vi "LDA_Beam_Alignment.vi"() -> ()   [LabVIEW 2010]
uses:
  Anemometry Sub Vis/Controls/Beam_Type.ctl
  Anemometry Sub Vis/Gen Trav/Traverse_cluster.ctl
  Anemometry Sub Vis/Gen Trav/Spacing.ctl
  Anemometry Sub Vis/Controls/Multi_run_mode.ctl
  Anemometry Sub Vis/Controls/User_Specific_mode.ctl
  Anemometry Sub Vis/Controls/Post_Process.ctl
  Anemometry Sub Vis/Controls/Tunnel_Coordinates.ctl
  Anemometry Sub Vis/Gen Trav/Trav_mode.ctl
  Anemometry Sub Vis/Globals/Trav_pos_global.vi
  Anemometry Sub Vis/Globals/Meas_global.vi
  Anemometry Sub Vis/Globals/Preference_global.vi
panel:
  in  "Beams to peak":bool[](array[boolean])=[TRUE, TRUE, TRUE, TRUE]
  out "Beam Names":string[](array[string])
  out "Probe is facing...":string
  out "In-Plane Roll (deg)":dbl
  out "Pitch (deg)":dbl
  out "Yaw (deg)":dbl
  out "Vp (Actual Probe dir. vect)":dbl[](array[numeric])
  in  "Mode":T1(ring)
  out "Values Out":dbl[][](array[numeric]) format="%.2f"
  out "Original Position":dbl[](array[numeric]) format="%.2f"
  in  "Traverse Position":dbl[](array[numeric])=[0.0, 0.0, 0.0] format="%.2f"
  out "Message":string
  in  "Go Back":bool
  in  "OK":bool
  in  "stop":bool
  in  "Working On":T2 items=["Green Unshifted", "Green Shifted", "Blue Unshifted", "Blue Shifted"]
  # "X                 Y              Z"
  # "X                 Y              Z          Power"
  # "Green Unshifted\nGreen Shifted\nBlue Unshifted\nBlue Shifted"
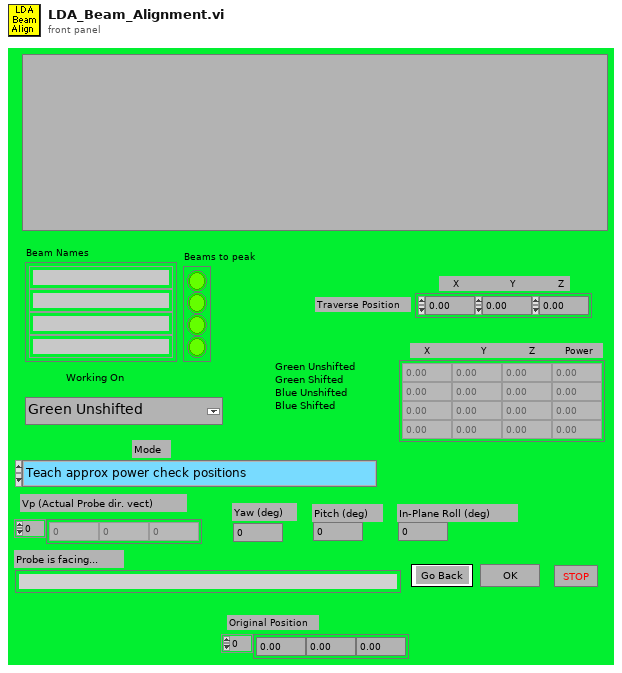
[diagram p1: front panel]
types:
  T1 = enum16{"Teach approx power check positions", "Hunt for optimum power check positions", "Check Beam powers now", "Peak up beam power using manipulators"}
  T2 = typedef "Beam_Type.ctl" = u16
  T3 = typedef "Traverse_cluster.ctl" = cluster{"Start X":dbl, "Start Y":dbl, "Start Z":dbl, "End X":dbl, "End Y":dbl, "End Z":dbl, "No. of pts.":i32, "Spacing":T4, "Filename":path, "Tunnel Speed":dbl, "Averaging time (min)":dbl, "Extra Commands":string, "Specific Arguments":string, "Emission Rate (l/min)":dbl, "Trace Gas Concentration (%)":dbl, "Density Ratio":string, "Comments":string, "Row No":i32, "Row Type Selector":T5, "Completion time":string, "Row Duration (mins)":dbl, "No. of Valid pts.":i32, "Meas Setup File":string}
  T4 = typedef "Spacing.ctl" = enum16{"Linear", "Log", "Gauss", "Specified", "N/A"}
  T5 = typedef "Multi_run_mode.ctl" = enum16{"Move Traverse Only", "Set Tunnel Speed Only", "Set Source Only", "Set Measurement Conditions", "Single Measurement", "Vertical Profile", "Lateral Profile", "Longitudinal Profile", "Explore Volume", "Multi-Axis Profile", "Auto Calibrate", "Meas Fast FID Bkgnd", "Check Beam Power", "Scanning Valve Measurement", "Run VI Named:", "Set ADAM Ch", "Wait (minutes)", "Send Message", "Synchronize With:", "Fall Back to this Row", "Turn Off Row Repeating", "Blank Row"}
  T6 = typedef "Tunnel_Coordinates.ctl" = enum16{"Work in Tunnel Coordinates", "Work in Model Coordinates"}
  T7 = typedef "User_Specific_mode.ctl" = enum16{"Check VI only", "Run VI"}
  T8 = typedef "Post_Process.ctl" = enum16{"Take New Data", "Post Process Raw Data File"}
  T9 = enum16{"Load setup from excel file", "Save setup to excel file"}
  T10 = enum16{"Load From Excel File", "Save to Excel File"}
  T11 = typedef "Trav_mode.ctl" = enum16{"Move traverse", "Read traverse position", "Teach Position"}
  T12 = typedef "LDA_Beam_Cluster.ctl" = cluster{"Vg1 (Green 1 dir. vect.)":dbl[], "Vg2  (Green 2 dir. vect.)":dbl[], "Vb1 (Blue 1 dir. vect.)":dbl[], "Vb2 (Blue 1 dir. vect.)":dbl[], "Porb (Orb XYZ posn. forced coplanar)":dbl[], "Porb (Orb XYZ posn. - allow skew)":dbl[], "Orb posn. uncertainty, +/- dx, dy, dz":dbl[], "Vp (Actual Probe dir. vect)":dbl[], "Yaw (deg)":dbl, "Pitch (deg)":dbl, "In-Plane Roll (deg)":dbl, "Beam Half Angle (deg)":dbl, "B1 Close P11":dbl[], "B1 Far P12":dbl[], "B2 Close P22":dbl[], "B2 Far P21":dbl[], "Projected Roll (deg)":dbl, "Green Velocity Vector":dbl[], "Blue Velocity Vector":dbl[], "Probe is facing....":string, "Calculation Method":string}
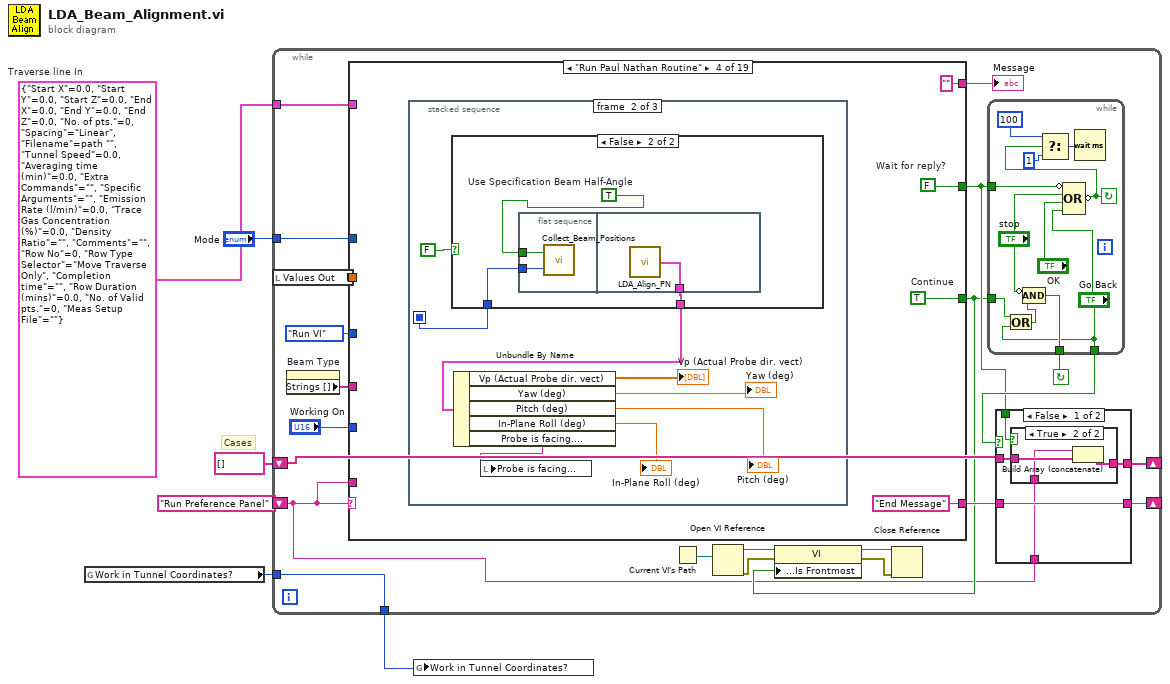
[diagram p0: block diagram]
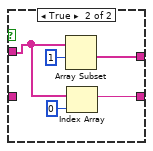
[diagram p3: hidden frame]
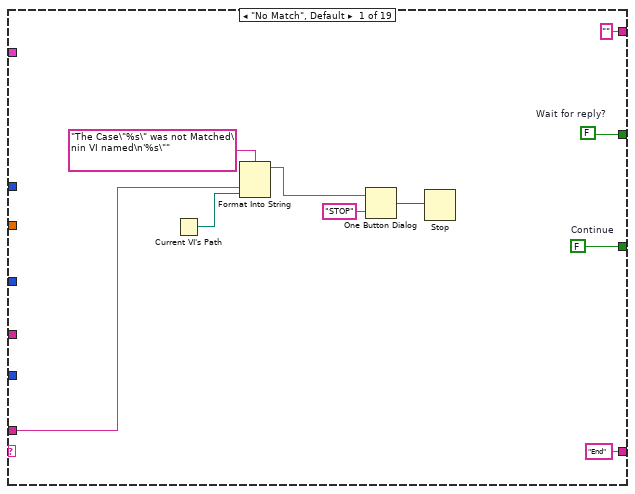
[diagram p4: hidden frame]
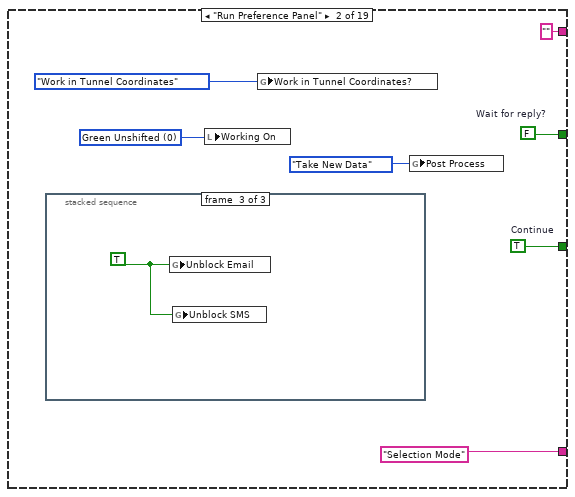
[diagram p5: hidden frame]
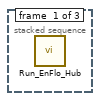
[diagram p6: hidden frame]
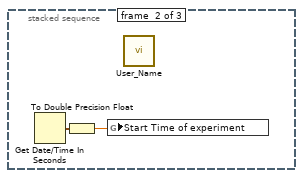
[diagram p7: hidden frame]
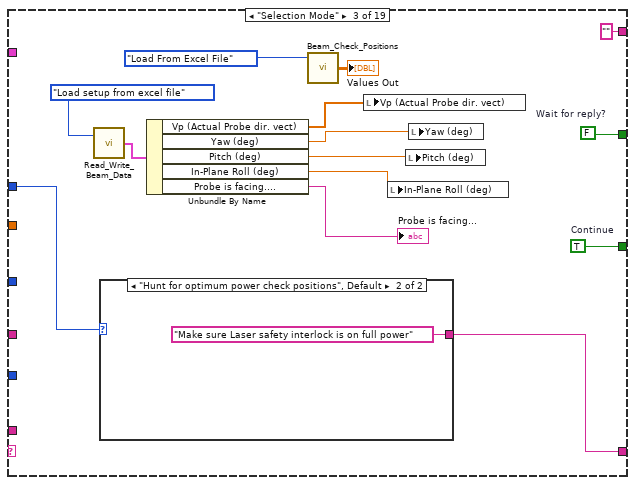
[diagram p8: hidden frame]
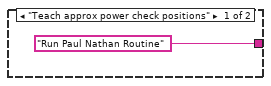
[diagram p9: hidden frame]
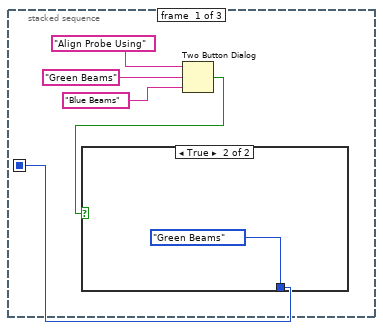
[diagram p10: hidden frame]
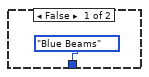
[diagram p11: hidden frame]
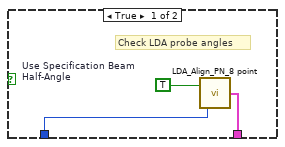
[diagram p12: hidden frame]
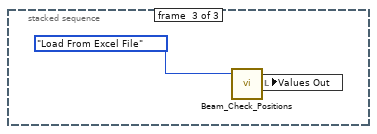
[diagram p13: hidden frame]
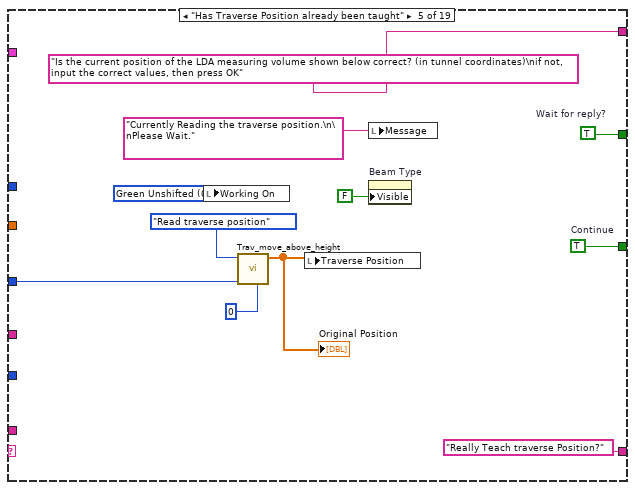
[diagram p14: hidden frame]
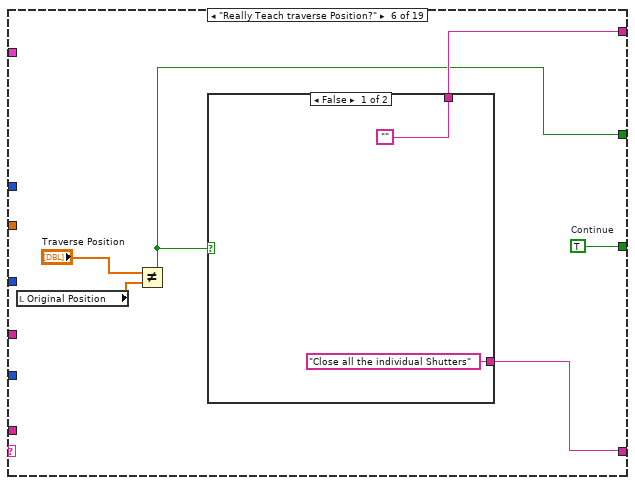
[diagram p15: hidden frame]
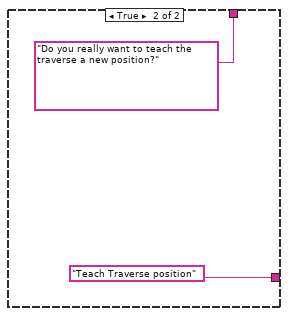
[diagram p16: hidden frame]
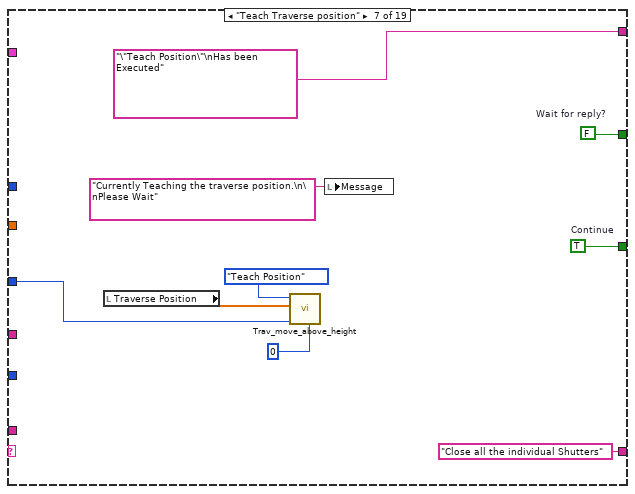
[diagram p17: hidden frame]
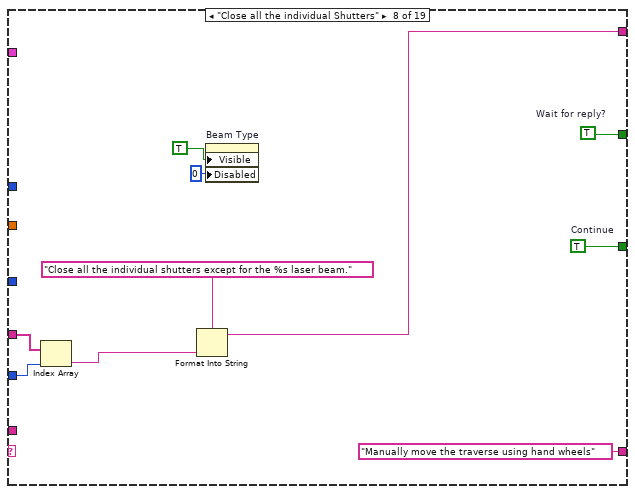
[diagram p18: hidden frame]
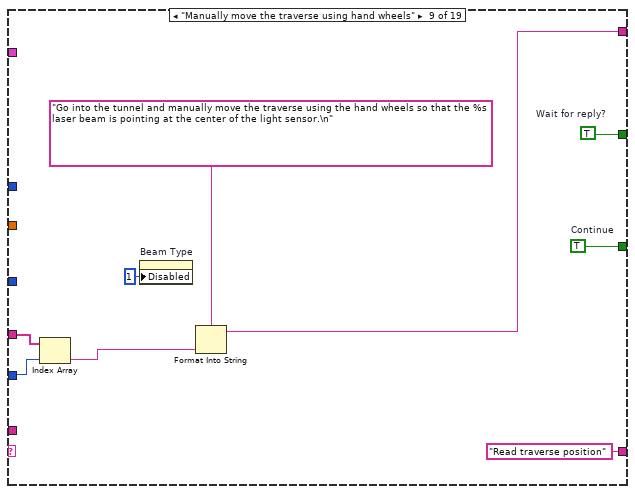
[diagram p19: hidden frame]
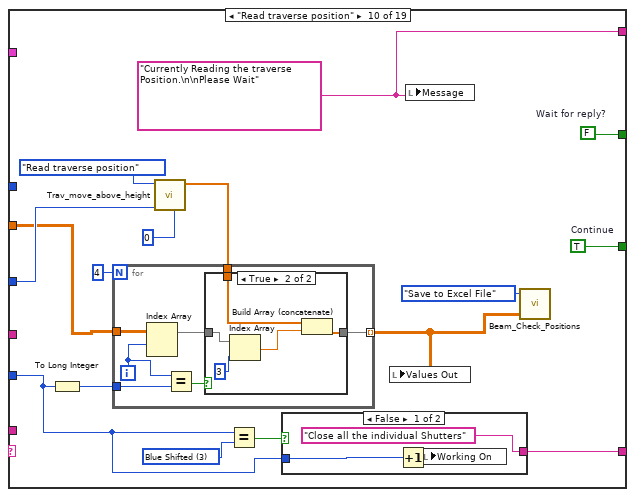
[diagram p20: hidden frame]
diagram:
  w3 = T3 {"Start X"=0.0, "Start Y"=0.0, "Start Z"=0.0, "End X"=0.0, "End Y"=0.0, "End Z"=0.0, "No. of pts."=0, "Spacing"=enum."Linear", "Filename"=path "", "Tunnel Speed"=0.0, "Averaging time (min)"=0.0, "Extra Commands"="", "Specific Arguments"="", "Emission Rate (l/min)"=0.0, "Trace Gas Concentration (%)"=0.0, "Density Ratio"="", "Comments"="", "Row No"=0, "Row Type Selector"=enum."Move Traverse Only", "Completion time"="", "Row Duration (mins)"=0.0, "No. of Valid pts."=0, "Meas Setup File"=""}  # Traverse line In
  # "Cases"
  n1 = global read "Trav_pos_global.vi" "Work in Tunnel Coordinates?"() -> (w1:T6)
  n2 = while {
    tunnel: w3 -> [w9]
    tunnel: "Mode" -> [w10]
    shift-left: string[] [] -> [w26]
    shift-right: [w25] -> _
    shift-left: "Run Preference Panel" -> [w8]
    shift-right: [w24] -> _
    tunnel: [w7] -> w2
    tunnel: w1 -> [w7]
    stop <- w28 continue-if-true
    n3 = local read "Values Out"() -> (w11:dbl[][])
    n4 = property on="Beam Type" class="Ring (strict)"() -> ("Strings []"=w13:string[])  [unwired: 2 in, 2 out]
    n5 = case shown="\"Run Paul Nathan Routine\"" w8 {
      tunnel: [w63 w70 w87 w93 w130 w136 w149 w159 w168 w184 w209 w219 w233 w259 w279 w283 w298 w306 w316] -> w14
      tunnel: ["End" "Selection Mode" w83 "End Message" "Really Teach traverse Position?" w131 "Close all the individual Shutters" "Manually move the traverse using hand wheels" "Read traverse position" w172 w203 "Hunt for optimum power check positions" "End Message" "End Message" "Read Beam Power" "Save measured beam Power" w290 "End Message" "End"] -> w23
      tunnel: [w62 w69 w86 w92 w129 w132 w148 w158 w167 w183 w208 w218 w234 w260 w278 w282 w297 w305 w315] -> w15
      tunnel: ["" "" "" "" "Is the current position of the LDA measuring volume shown below correct? (in tunnel coordinates)\nif not, input the correct values, then press OK" w135 "\"Teach Position\"\nHas been Executed" w152 w161 w169 "Make sure the Laser safety interlock is on full power and all the shutters are open." "Please select which beams you would like to hunt for optimum power check positions for by pressing the green buttons." "" "" w265 w281 w289 "Now open all the individual shutters so all four beam are showing." w309] -> w22
      tunnel: User_Specific_mode."Run VI" ("Simulate/Run") -> [_ _ _ _ w125 _ w144 _ _ w180 _ _ _ _ w275 _ _ _ _]
      tunnel: w13 -> [_ _ _ _ _ _ _ w157 w164 _ w206 w214 w222 _ w270 _ w286 _ _]
      tunnel: "Working On" -> [_ _ _ _ _ _ _ w156 w163 w171 w205 _ _ _ w269 _ w287 _ _]
      tunnel: w11 -> [_ _ _ _ _ _ _ _ _ w170 _ _ _ _ w268 _ w295 _ _]
      tunnel: w10 -> [_ _ w84 _ _ _ _ _ _ _ w204 _ _ _ _ _ _ _ w312]
      tunnel: w9 -> [_ _ _ _ _ _ _ _ _ _ _ _ _ w257 _ _ _ _ _]
      tunnel: w8 -> [w54 _ _ _ _ _ _ _ _ _ _ _ _ _ _ _ _ _ _]
      frame "No Match", Default {
        w62 = FALSE  # Wait for reply?
        w63 = FALSE  # Continue
        n6 = Current VI's Path() -> (path=w55:path)
        n7 = Format Into String(format string="The Case\"%s\" was not Matched\nin VI named\n'%s\"" ("Format String"), w54, w55) -> (resulting string=w58:string)  [unwired: 2 in, 1 out]
        n8 = One Button Dialog(message=w58, button name ("OK")="STOP") -> (true=w56:bool)
        n9 = Stop(stop? (T)=w56) -> ()
      }
      frame "Run Preference Panel" {
        w67 = T2 0 items=["Green Unshifted", "Green Shifted", "Blue Unshifted", "Blue Shifted"] ("Beam Type")
        w69 = FALSE  # Wait for reply?
        w70 = TRUE  # Continue
        n10 = stacked-sequence {
          frame #0 {
            n11 = call "Run_EnFlo_Hub.vi"() -> ()  [unwired: 8 out]
          }
          frame #1 {
            n12 = Get Date/Time In Seconds() -> (seconds since 1Jan1904=w72:timestamp)
            n13 = To Double Precision Float(number=w72) -> (double precision float=w71:dbl)
            n14 = global write "Meas_global.vi" "Start Time of experiment"(w71) -> ()
            n15 = call "User_Name.vi"() -> ()  [unwired: 1 out]
          }
          frame #2 {
            w73 = TRUE
            n16 = global write "Preference_global.vi" "Unblock Email"(w73) -> ()
            n17 = global write "Preference_global.vi" "Unblock SMS"(w73) -> ()
          }
        }
        n18 = local write "Working On"(w67) -> ()
        n19 = global write "Trav_pos_global.vi" "Work in Tunnel Coordinates?"(Tunnel_Coordinates."Work in Tunnel Coordinates" ("Work in Tunnel Coordinates?")) -> ()
        n20 = global write "Meas_global.vi" "Post Process"(Post_Process."Take New Data" ("Post Process")) -> ()
      }
      frame "Selection Mode" {
        w86 = FALSE  # Wait for reply?
        w87 = TRUE  # Continue
        n21 = call "Read_Write_Beam_Data.vi"("Mode"=T9."Load setup from excel file") -> ("Beam Data Out"=w75:T12)  [unwired: 1 in]
        n22 = case shown="\"Hunt for optimum power check positions\", Default" w84 {
          tunnel: ["Run Paul Nathan Routine" "Make sure Laser safety interlock is on full power"] -> w83
          frame "Teach approx power check positions" {
          }
          frame "Hunt for optimum power check positions", Default {
          }
        }
        n23 = Unbundle By Name(w75) -> ("Vp (Actual Probe dir. vect)"=w80:dbl[], "Yaw (deg)"=w77:dbl, "Pitch (deg)"=w78:dbl, "In-Plane Roll (deg)"=w79:dbl, "Probe is facing...."=→"Probe is facing...":string)
        n24 = call "Beam_Check_Positions.vi"("Mode"=T10."Load From Excel File") -> ("Values Out"=→"Values Out":dbl[][])  [unwired: 1 in, 1 out]
        n25 = local write "Vp (Actual Probe dir. vect)"(w80) -> ()
        n26 = local write "In-Plane Roll (deg)"(w79) -> ()
        n27 = local write "Pitch (deg)"(w78) -> ()
        n28 = local write "Yaw (deg)"(w77) -> ()
      }
      frame "Run Paul Nathan Routine" {
        w92 = FALSE  # Wait for reply?
        w93 = TRUE  # Continue
        n29 = stacked-sequence {
          seq-local: [w94 _ _] -> [_ w102 _]
          frame #0 {
            n30 = Two Button Dialog(message="Align Probe Using", 1:"Blue Beams" ("F button name (\"Cancel\")"), 2:"Green Beams" ("T button name (\"OK\")")) -> (T button?=w95:bool)
            n31 = case shown="True" w95 {
              tunnel: [enum16{"Green Beams", "Blue Beams"}."Blue Beams" ("Align Probe Using") enum16{"Green Beams", "Blue Beams"}."Green Beams" ("Align Probe Using")] -> w94
              frame False {
              }
              frame True {
              }
            }
          }
          frame #1 {
            n32 = case shown="False" FALSE ("Case Constant\n(See Context Help)") {
              tunnel: [w110 w112] -> w108
              tunnel: w102 -> [w109 w114]
              frame True {
                w111 = TRUE  # Use Specification Beam Half-Angle
                # "Check LDA probe angles"
                n33 = call "LDA_Align_PN_8 point.vi"("Align Probe Using"=w109, "Use Specification Beam Half-Angle"=w111) -> ("Beam Data"=w110:T12)
              }
              frame False {
                w113 = TRUE  # Use Specification Beam Half-Angle
                n34 = flat-sequence {
                  tunnel: w114 -> [w116]
                  tunnel: w113 -> [w115]
                  tunnel: [w117] -> w112
                  frame #0 {
                    n35 = call "Collect_Beam_Positions.vi"("Align Probe Using"=w116, "Use Specification Beam Half-Angle"=w115) -> ()  [unwired: 1 out]
                  }
                  frame #1 {
                    n36 = call "LDA_Align_PN.vi"() -> ("Beam Data"=w117:T12)  [unwired: 2 in]
                  }
                }
              }
            }
            n37 = Unbundle By Name(w108) -> ("Vp (Actual Probe dir. vect)"=→"Vp (Actual Probe dir. vect)":dbl[], "Yaw (deg)"=→"Yaw (deg)":dbl, "Pitch (deg)"=→"Pitch (deg)":dbl, "In-Plane Roll (deg)"=→"In-Plane Roll (deg)":dbl, "Probe is facing...."=w103:string)
            n38 = local write "Probe is facing..."(w103) -> ()
          }
          frame #2 {
            n39 = call "Beam_Check_Positions.vi"("Mode"=T10."Load From Excel File") -> ("Values Out"=w118:dbl[][])  [unwired: 1 in, 1 out]
            n40 = local write "Values Out"(w118) -> ()
          }
        }
      }
      frame "Has Traverse Position already been taught" {
        w123 = T2 0 items=["Green Unshifted", "Green Shifted", "Blue Unshifted", "Blue Shifted"] ("Beam Type")
        w129 = TRUE  # Wait for reply?
        w130 = TRUE  # Continue
        n41 = local write "Working On"(w123) -> ()
        n42 = call "Trav_move_above_height.vi"("Currently on Point"=0, "Simulate/Run"=w125, "Mode"=Trav_mode."Read traverse position") -> ("Trav Position achieved"=w124:dbl[])  [unwired: 4 in, 4 out]
        "Original Position" <- w124
        n43 = local write "Traverse Position"(w124) -> ()
        n44 = local write "Message"("Currently Reading the traverse position.\n\nPlease Wait." ("Message")) -> ()
        n45 = property on="Beam Type" class="Ring (strict)"("Visible"=FALSE ("Write Attribute")) -> ()  [unwired: 2 in, 2 out]
      }
      frame "Really Teach traverse Position?" {
        w136 = TRUE  # Continue
        n46 = local read "Original Position"() -> (w134:dbl[])
        n47 = Not Equal?(x="Traverse Position", y=w134) -> (x != y?=w132:bool)
        n48 = case shown="False" w132 {
          tunnel: ["" "Do you really want to teach the traverse a new position?"] -> w135
          tunnel: ["Close all the individual Shutters" "Teach Traverse position"] -> w131
          frame False {
          }
          frame True {
          }
        }
      }
      frame "Teach Traverse position" {
        w148 = FALSE  # Wait for reply?
        w149 = TRUE  # Continue
        n49 = local read "Traverse Position"() -> (w143:dbl[])
        n50 = call "Trav_move_above_height.vi"("Currently on Point"=0, "Simulate/Run"=w144, "New Position"=w143, "Mode"=Trav_mode."Teach Position") -> ()  [unwired: 3 in, 5 out]
        n51 = local write "Message"("Currently Teaching the traverse position.\n\nPlease Wait" ("Message")) -> ()
      }
      frame "Close all the individual Shutters" {
        w158 = TRUE  # Wait for reply?
        w159 = TRUE  # Continue
        n52 = Index Array(array=w157, index=w156) -> (element=w155:string)
        n53 = Format Into String(format string="Close all the individual shutters except for the %s laser beam.", w155) -> (resulting string=w152:string)  [unwired: 2 in, 1 out]
        n54 = property on="Beam Type" class="Ring (strict)"("Visible"=TRUE ("Write Attribute"), "Disabled"=u8 0 ("Write Attribute")) -> ()  [unwired: 2 in, 2 out]
      }
      frame "Manually move the traverse using hand wheels" {
        w167 = TRUE  # Wait for reply?
        w168 = TRUE  # Continue
        n55 = Index Array(array=w164, index=w163) -> (element=w165:string)
        n56 = property on="Beam Type" class="Ring (strict)"("Disabled"=u8 1 ("Write Attribute")) -> ()  [unwired: 2 in, 2 out]
        n57 = Format Into String(format string="Go into the tunnel and manually move the traverse using the hand wheels so that the %s laser beam is pointing at the center of the light sensor.\n", w165) -> (resulting string=w161:string)  [unwired: 2 in, 1 out]
      }
      frame "Read traverse position" {
        w174 = T2 3 items=["Green Unshifted", "Green Shifted", "Blue Unshifted", "Blue Shifted"] ("Beam Type")
        w169 = "Currently Reading the traverse Position.\n\nPlease Wait"
        w183 = FALSE  # Wait for reply?
        w184 = TRUE  # Continue
        n58 = To Long Integer(number=w171) -> (32bit integer=w179:i32)
        n59 = call "Trav_move_above_height.vi"("Currently on Point"=0, "Simulate/Run"=w180, "Mode"=Trav_mode."Read traverse position") -> ("Trav Position achieved"=w178:dbl[])  [unwired: 4 in, 4 out]
        n60 = for {
          N: 4 -> [_]
          tunnel: w170 -> [w195]
          tunnel: w179 -> [w193]
          tunnel: [w191] -> w175 mode=indexing
          tunnel: w178 -> [w189]
          i -> [w194]
          n61 = Index Array(array=w195, index (row)=w194) -> (element=w190:dbl[])  [unwired: 1 in]
          n62 = Equal?(x=w194, y=w193) -> (x = y?=w192:bool)
          n63 = case shown="True" w192 {
            tunnel: [w196 w199] -> w191
            tunnel: w190 -> [w196 w201]
            tunnel: w189 -> [_ w197]
            frame False {
            }
            frame True {
              n64 = Index Array(array=w201, index=3 ("Index")) -> (element=w198:dbl)
              n65 = Build Array (concatenate)(w197, w198) -> (w199:dbl[])
            }
          }
        }
        n66 = Equal?(x=w171, y=w174) -> (x = y?=w173:bool)
        n67 = case shown="False" w173 {
          tunnel: ["Close all the individual Shutters" "Open all individual laser shutters again"] -> w172
          tunnel: w171 -> [w186 _]
          frame False {
            n68 = Increment(x=w186) -> (x+1=w187:T2)
            n69 = local write "Working On"(w187) -> ()
          }
          frame True {
          }
        }
        n70 = local write "Values Out"(w175) -> ()
        n71 = local write "Message"(w169) -> ()
        n72 = call "Beam_Check_Positions.vi"("Values"=w175, "Mode"=T10."Save to Excel File") -> ()  [unwired: 2 out]
      }
      frame "Make sure Laser safety interlock is on full power" {
        w208 = TRUE  # Wait for reply?
        w209 = TRUE  # Continue
        n73 = Index Array(array=w206, index=w205) -> ()  [unwired: 1 out]
        n74 = property on="Beam Type" class="Ring (strict)"("Disabled"=u8 1 ("Write Attribute")) -> ()  [unwired: 2 in, 2 out]
        n75 = case shown="\"Hunt for optimum power check positions\"" w204 {
          tunnel: ["Has Traverse Position already been taught" "Find Peak for which beams?" "Check Beam powers now" "Move Traverse to next Meas position"] -> w203
          frame "Teach approx power check positions" {
          }
          frame "Hunt for optimum power check positions" {
          }
          frame "Check Beam powers now" {
          }
          frame "Peak up beam power using manipulators" {
          }
        }
      }
      frame "Find Peak for which beams?" {
        w218 = TRUE  # Wait for reply?
        w219 = TRUE  # Continue
        n76 = property on="Beam Type" class="Ring (strict)"("Disabled"=u8 1 ("Write Attribute")) -> ()  [unwired: 2 in, 2 out]
        "Beam Names" <- w214
      }
      frame "Hunt for optimum power check positions" {
        w234 = FALSE  # Wait for reply?
        w233 = TRUE  # Continue
        w239 = T3 {"Start X"=0.0, "Start Y"=0.0, "Start Z"=0.0, "End X"=0.0, "End Y"=0.0, "End Z"=0.0, "No. of pts."=0, "Spacing"=enum."Linear", "Filename"=path "", "Tunnel Speed"=0.0, "Averaging time (min)"=0.0, "Extra Commands"="", "Specific Arguments"="", "Emission Rate (l/min)"=0.0, "Trace Gas Concentration (%)"=0.0, "Density Ratio"="", "Comments"="", "Row No"=0, "Row Type Selector"=enum."Move Traverse Only", "Completion time"="", "Row Duration (mins)"=0.0, "No. of Valid pts."=0, "Meas Setup File"=""}  # Traverse line In
        w225 = 0.85 ("y")
        n77 = local read "Vp (Actual Probe dir. vect)"() -> (w231:dbl[])
        n78 = for {
          shift-right: [w243] -> w221
          shift-left: "; " -> [w242]
          tunnel: "Beams to peak" -> [w244] mode=indexing
          tunnel: w222 -> [w241] mode=indexing
          n79 = case shown="True" w244 {
            tunnel: [w245 w249] -> w243
            tunnel: w242 -> [w245 w248]
            tunnel: w241 -> [_ w247]
            frame False {
            }
            frame True {
              n80 = Concatenate Strings(w248, w247, ";  " ("string")) -> (w249:string)
            }
          }
        }
        n81 = Absolute Value(x=w231) -> (abs(x)=w230:dbl[])
        n82 = Array To Cluster(array=w230) -> (cluster=w229:cluster{"[0]":dbl, "[1]":dbl, "[2]":dbl})
        n83 = Unbundle(w229) -> ("[0]"=w228:dbl, "[1]"=w226:dbl)  [unwired: 1 out]
        n84 = Greater?(x=w228, y=w225) -> (0:w227:bool)
        n85 = case shown="True" w227 {
          tunnel: [w253 "X Axis Fixed"] -> w240
          tunnel: w226 -> [w252 _]
          tunnel: w225 -> [w251 _]
          frame False {
            n86 = Greater?(x=w252, y=w251) -> (0:w250:bool)
            n87 = case shown="False" w250 {
              tunnel: ["Z Axis Fixed" "Y Axis Fixed"] -> w253
              frame False {
              }
              frame True {
              }
            }
          }
          frame True {
          }
        }
        n88 = Concatenate Strings("First Argument;" ("string"), w240, w221) -> (w238:string)
        n89 = Bundle By Name(cluster=w239, "Specific Arguments"=w238) -> (w237:T3)
        n90 = call "Find_Beam_Max_Pos.vi"("Mode"=User_Specific_mode."Run VI", "Traverse line In"=w237) -> ()  [unwired: 4 out]
      }
      frame "Check Beam powers now" {
        w260 = FALSE  # Wait for reply?
        w259 = TRUE  # Continue
        n91 = call "Check_Beam_Powers.vi"("Mode"=User_Specific_mode."Run VI", "Traverse line In"=w257) -> ()  [unwired: 4 out]
      }
      frame "Move Traverse to next Meas position" {
        w278 = FALSE  # Wait for reply?
        w279 = TRUE  # Continue
        n92 = Index Array(array=w270, index=w269) -> (element=w263:string)
        n93 = Format Into String(format string="The %s laser beam should now be hitting the light sensor. Please Peak up this beam to achieve the maximum output", w263) -> (resulting string=w265:string)  [unwired: 2 in, 1 out]
        n94 = Format Into String(format string="Currently moving Traverse.\n\nThe %s Laser Beam should soon be hitting the light sensor.\n\nPlease Wait", w263) -> (resulting string=w267:string)  [unwired: 2 in, 1 out]
        n95 = call "PM100D_Plot_ph.vi"("Beam Name"=w263) -> ()  [unwired: 1 out]
        n96 = Index Array(array=w268, index (row)=w269) -> (element=w274:dbl[])  [unwired: 1 in]
        n97 = local write "Message"(w267) -> ()
        n98 = Array Subset(array=w274, length=3 ("Array Length")) -> (w272:dbl[])  [unwired: 1 in]
        n99 = call "Trav_move_above_height.vi"("Currently on Point"=0, "Simulate/Run"=w275, "New Position"=w272, "Mode"=Trav_mode."Move traverse") -> ()  [unwired: 3 in, 5 out]
      }
      frame "Read Beam Power" {
        w281 = "Currently Reading the Beam Power\n\nPlease Wait"
        w282 = FALSE  # Wait for reply?
        w283 = TRUE  # Continue
        n100 = local write "Message"(w281) -> ()
      }
      frame "Save measured beam Power" {
        w292 = T2 3 items=["Green Unshifted", "Green Shifted", "Blue Unshifted", "Blue Shifted"] ("Beam Type")
        w289 = "Writing Beam Power to file"
        w297 = FALSE  # Wait for reply?
        w298 = TRUE  # Continue
        n101 = Index Array(array=w286, index=w287) -> (element=w285:string)
        n102 = Equal?(x=w287, y=w292) -> (x = y?=w291:bool)
        n103 = call "PM100D_Single_Value_ph.vi"("Averaging Period (s)"=3.0, "Beam Name"=w285) -> ("Light Power mW"=w288:dbl)  [unwired: 1 out]
        n104 = case shown="False" w291 {
          tunnel: ["Move Traverse to next Meas position" "End Message"] -> w290
          tunnel: w287 -> [w301 _]
          frame False {
            n105 = Increment(x=w301) -> (x+1=w300:T2)
            n106 = local write "Working On"(w300) -> ()
          }
          frame True {
          }
        }
        n107 = Replace Array Subset(array=w295, new element=w288, index (row)=w287, index (col)=3 ("Index")) -> (w293:dbl[][])
        n108 = local write "Message"(w289) -> ()
        n109 = local write "Values Out"(w293) -> ()
        n110 = call "Beam_Check_Positions.vi"("Values"=w293, "Mode"=T10."Save to Excel File") -> ()  [unwired: 2 out]
      }
      frame "Open all individual laser shutters again" {
        w305 = TRUE  # Wait for reply?
        w306 = TRUE  # Continue
      }
      frame "End Message" {
        w315 = FALSE  # Wait for reply?
        w316 = FALSE  # Continue
        n111 = property on="Mode" class="Enum (strict)"() -> ("Strings []"=w313:string[])  [unwired: 2 in, 2 out]
        n112 = Index Array(array=w313, index=w312) -> (element=w311:string)
        n113 = Format Into String(format string="%s\nhas now been completed" ("Format String"), w311) -> (resulting string=w309:string)  [unwired: 2 in, 1 out]
        n114 = call "Beam_Check_Positions.vi"("Mode"=T10."Load From Excel File") -> ("Values Out"=w307:dbl[][])  [unwired: 1 in, 1 out]
        n115 = local write "Values Out"(w307) -> ()
      }
    }
    "Message" <- w22
    n116 = Current VI's Path() -> (path=w20:path)
    n117 = Open VI Reference(vi path=w20) -> (vi reference=w19:refnum<vi>, error out=w18:errorcluster)  [unwired: 1 in, 4 out]
    n118 = property class="VI"(reference=w19, error in=w18, "Front Panel Window:Is Frontmost"=w14) -> (reference out=w17:refnum<vi>, error out=w16:errorcluster)
    n119 = Close Reference(reference=w17, error in (no error)=w16) -> ()  [unwired: 1 out]
    n120 = while {
      tunnel: ["Go Back"] -> w27
      tunnel: [w36] -> w28
      tunnel: w14 -> [w35]
      tunnel: w15 -> [w38]
      stop <- w32 continue-if-true
      n121 = Or(x=w35, y="Go Back") -> (x .or. y?=w33:bool)
      n122 = Compound Arithmetic op=AND(invert "stop", w33) -> (w36:bool)
      n123 = Compound Arithmetic op=OR(invert w38, "stop", "OK", "Go Back") -> (invert w32:bool)
      n124 = Select(t=u32 100 ("millisecond timer value"), s=w32, f=u32 1) -> (s? t:f=w29:u32)
      n125 = Wait (ms)(milliseconds to wait=w29) -> ()  [unwired: 1 out]
    }
    n126 = case shown="False" w27 {
      tunnel: w26 -> [w44 w49]
      tunnel: [w43 w50] -> w25
      tunnel: w8 -> [w41 _]
      tunnel: [w42 w51] -> w24
      tunnel: w23 -> [w42 _]
      tunnel: w15 -> [w40 _]
      frame False {
        n127 = case shown="True" w40 {
          tunnel: w44 -> [w45 w48]
          tunnel: [w45 w47] -> w43
          tunnel: w41 -> [_ w46]
          frame False {
          }
          frame True {
            n128 = Build Array (concatenate)(w46, w48) -> (w47:string[])
          }
        }
      }
      frame True {
        n129 = Array Subset(array=w49, index=1 ("Array Index")) -> (w50:string[])  [unwired: 1 in]
        n130 = Index Array(array=w49, index=0 ("Index")) -> (element=w51:string)
      }
    }
  }
  n131 = global write "Trav_pos_global.vi" "Work in Tunnel Coordinates?"(w2) -> ()
